vi "UltrasonicAnemoInputScale.vi"(1 "Wind Speed Ofst (m/s)":dbl, 2 "Wind Speed Scale (m/s per m/s)":dbl, 3 "Raw Wind Speed (m/s)":dbl) -> (0 "Wind Speed (m/s)":dbl)   [LabVIEW 2018]
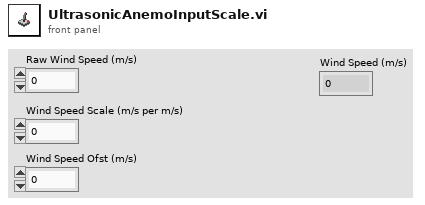
[diagram p1: front panel]
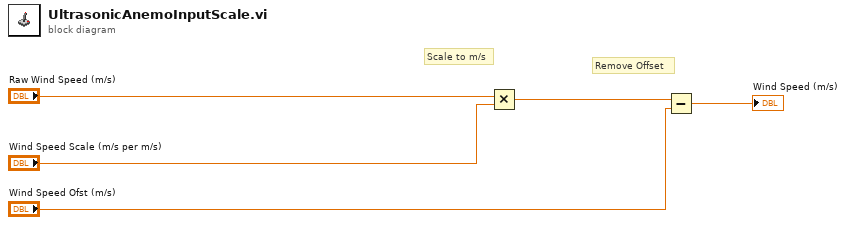
[diagram p0: block diagram]
diagram:
  # "Scale to m/s"
  # "Remove Offset"
  n1 = Multiply(x="Raw Wind Speed (m/s)", y="Wind Speed Scale (m/s per m/s)") -> (x*y=w2:dbl)
  n2 = Subtract(x=w2, y="Wind Speed Ofst (m/s)") -> (x-y=→"Wind Speed (m/s)":dbl)
